vi "Report to Subpanel.vi"(2 "error in (no error)":errorcluster, 3 "State":variant, 4 "controller in":refnum<class "Generic Plugin.lvclass">) -> (0 "error out":errorcluster, 1 "controller out":refnum<class "Generic Plugin.lvclass">)   [LabVIEW 2020, in "Generic Plugin.lvclass"]
uses:
  Generic Plugin.lvclass
  Generic Plugin.lvclass/Generic Plugin.ctl
  Sub VIs/Message Queue/test Message Queue.lvlib
  Sub VIs/Message Queue/Enqueue Message (Single).vi
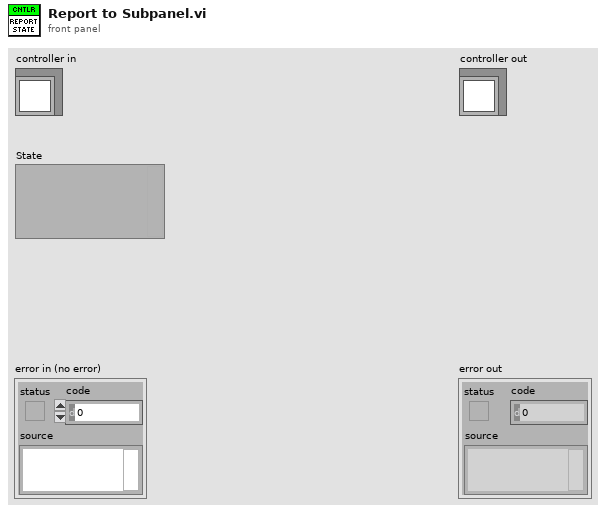
[diagram p1: front panel]
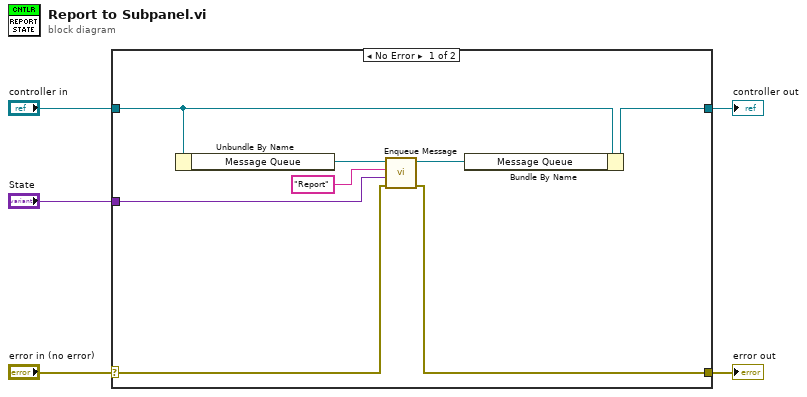
[diagram p0: block diagram]
diagram:
  n1 = case shown="No Error" "error in (no error)" {
    selector: "error in (no error)" -> [w7 w15]
    tunnel: [w6 w15] -> w4
    tunnel: [w11 w14] -> w2
    tunnel: "controller in" -> [w13 w14]
    tunnel: "State" -> [w8 _]
    frame No Error {
      n2 = Unbundle By Name(w13) -> ("Message Queue"=w12:refnum<queue>)
      n3 = call-poly "Enqueue Message.vi"("error in (no error)"=w7, "Message Data"=w8, "Message"="Report", "Message Queue"=w12) -> ("error out"=w6:errorcluster, "dup Message Queue"=w10:refnum<queue>)  [unwired: 6 in]
      n4 = Bundle By Name(cluster=w13, "Message Queue"=w10) -> (w11:refnum<class "Generic Plugin.lvclass">)
    }
    frame Error {
    }
  }
  "error out" <- w4
  "controller out" <- w2
